vi "WaveFormDeviation.vi"() -> ()   [LabVIEW 2023]
uses:
  <vilib>/Utility/file.llb/Read Delimited Spreadsheet (DBL).vi
panel:
  out "Waveform Chart":i64[][](graph)
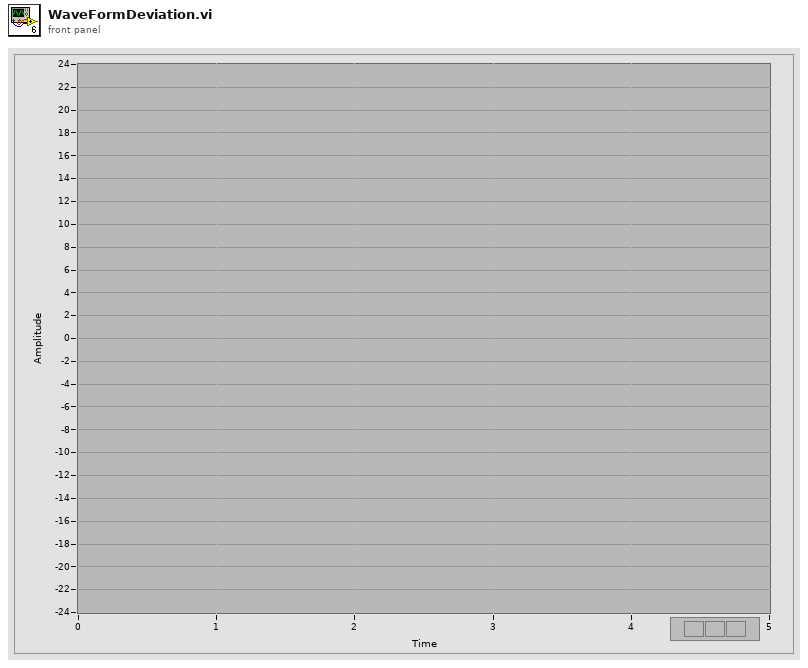
[diagram p1: front panel]
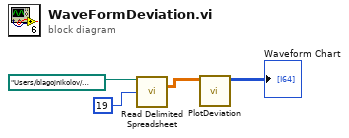
[diagram p0: block diagram]
diagram:
  n1 = call-poly <vilib>:"Read Delimited Spreadsheet.vi"("file path (dialog if empty)"=path "/Users/blagojnikolov/Desktop/@tmp/checkRes.txt", "start of read offset (chars.:0)"=19) -> ("all rows"=w2:dbl[][])  [unwired: 8 in, 5 out]
  n2 = call "PlotDeviation.vi"("Array"=w2) -> ("Waveform Chart"=→"Waveform Chart":i64[][])  [unwired: 7 in, 3 out]
